vi "UserVars-Substitute Into Expression.vi"(0 "Expression In":string, 7 "UserVars":T1[](array[typedef]), 11 "error in (no error)":errorcluster) -> (4 "Expression Out":string, 6 "Parsed Formula":cluster{"Table":i32[][], "Y Values":dbl[]} {"Y Values" format="%.2f"}, 15 "error out":errorcluster)   [LabVIEW 2020]
uses:
  User Variable.ctl
  <vilib>/gmath/NI_Gmath.lvlib
panel:
  # "operator"
  # "register1"
  # "register2"
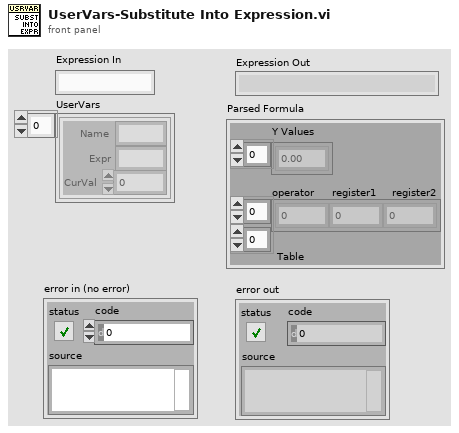
[diagram p1: front panel]
types:
  T1 = typedef "User Variable.ctl" = cluster{"Name":string, "Expr":string, "CurVal":dbl}
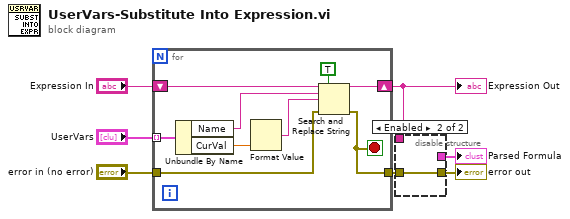
[diagram p0: block diagram]
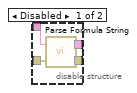
[diagram p2: hidden frame]
diagram:
  n1 = for {
    tunnel: "UserVars" -> [w16] mode=indexing
    shift-right: [w11] -> w2
    shift-left: "Expression In" -> [w15]
    tunnel: "error in (no error)" -> [w9]
    tunnel: [w8] -> w4
    stop <- w8 stop-if-true
    n2 = Unbundle By Name(w16) -> ("Name"=w14:string, "CurVal"=w13:dbl)
    n3 = Format Value(value (0)=w13) -> (output string=w12:string)  [unwired: 2 in]
    n4 = Search and Replace String(replace all?=TRUE ("replace all? (F)"), input string=w15, search string=w14, replace string=w12, error in=w9) -> (result string=w11:string, error out=w8:errorcluster)  [unwired: 3 in, 2 out]
  }
  "Expression Out" <- w2
  n5 = disable-structure shown="Enabled" {
    disable-tunnel: w4 -> [w20 w21]
    disable-tunnel: [w19 w21] -> w3
    disable-tunnel: w2 -> [w18 _]
    disable-tunnel: [w17 _] -> w1
    frame Disabled {
      n6 = call <vilib>:"Parse Formula String.vi"("error in (no error)"=w20, "formula"=w18) -> ("error out"=w19:errorcluster, "Parsed Formula"=w17:cluster{"Table":i32[][], "Y Values":dbl[]})
    }
    frame Enabled {
    }
  }
  "error out" <- w3
  "Parsed Formula" <- w1
